vi "Autonomous Independent.vi"   [LabVIEW 2019]
doc: "This VI is called when autonomous begins, and will automatically be terminated when autonomous ends. You can carry out timed or sensor driven robot movement independently without needing to return to the caller."
uses:
  <vilib>/Rock Robotics/WPI/Utilities/WPI_GetSetVariantRefNum.vi
  <vilib>/Rock Robotics/Network Tables/NT Read String.vi
  <vilib>/Rock Robotics/Network Tables/NT Write Numeric Array.vi
panel:
  # "Be sure to right-click and choose Data Operations>>Make Current Value default if you want to save the array values with the VI"
types:
  T1 = typedef "WPI_JoystickDevRef.ctl" = cluster{"Device":T2}
  T2 = typedef "WPI_JoystickDeviceEnum.ctl" = enum16{"USB 0", "USB 1", "USB 2", "USB 3", "USB 4", "USB 5"}
  T3 = typedef "WPI_RobotDriveDevRef.ctl" = cluster{"DevStatus":errorcluster, "Motors[]":T4[], "Square Inputs":bool, "Max Output":dbl}
  T4 = typedef "WPI_MotorControlDeviceRef.ctl" = cluster{"DeviceStatus":errorcluster, "Type":T5, "PWM":cluster{"PWM Channel":T6, "DeadBand":T7}, "CAN":cluster{"Device Number":u8, "SetOutput VI Ref":variant, "GetOutput VI Ref":variant, "Enable VI Ref":variant, "Disable VI Ref":variant, "Data":variant}, "Invert":bool, "DIO PWM":cluster{"PWM \"Enable\" Channel":T6, "DIOChannel":T8, "PWM Rate":dbl}}
  T5 = typedef "WPI_MotorControlType.ctl" = enum16{"PWM", "CAN", "DIO PWM"}
  T6 = typedef "FPGA_DIOPWMChannel.ctl" = enum8{"PWM 0", "PWM 1", "PWM 2", "PWM 3", "PWM 4", "PWM 5", "PWM 6", "PWM 7", "PWM 8", "PWM 9", "PWM MXP 0", "PWM MXP 1", "PWM MXP 2", "PWM MXP 3", "PWM MXP 4", "PWM MXP 5", "PWM MXP 6", "PWM MXP 7", "PWM MXP 8", "PWM MXP 9", "Invalid"}
  T7 = typedef "WPI_PWMDeadband.ctl" = cluster{"Name":string, "maxPositivePwm":i32, "minPositivePwm":i32, "centerPwm":i32, "maxNegativePwm":i32, "minNegativePwm":i32, "angularRange":u16}
  T8 = typedef "FPGA_DIOChannel.ctl" = enum8{"DIO 0", "DIO 1", "DIO 2", "DIO 3", "DIO 4", "DIO 5", "DIO 6", "DIO 7", "DIO 8", "DIO 9", "DIO MXP 0", "DIO MXP 1", "DIO MXP 2", "DIO MXP 3", "DIO MXP 4", "DIO MXP 5", "DIO MXP 6", "DIO MXP 7", "DIO MXP 8", "DIO MXP 9", "DIO MXP 10", "DIO MXP 11", "DIO MXP 12", "DIO MXP 13", "DIO MXP 14", "DIO MXP 15", "SPI Port CS1", "SPI Port CS2", "SPI Port CS3", "SPI Port MISO", "SPI Port MOSI", "Invalid"}
  T9 = typedef "WPI_GyroDevRef.ctl" = cluster{"DevStatus":errorcluster, "Analog Channel":T10, "Gain (VoltsPerDegree/Second)":dbl, "Gyro Type":enum16{"Analog", "XRS450"}, "Handle":i32, "SPI Bus":T11, "Device Found":bool, "Sample Rate":dbl, "Calibrate On Open":bool, "Offset":dbl}
  T10 = typedef "FPGA_AIChannel.ctl" = enum8{"AI 0", "AI 1", "AI 2", "AI 3", "AI MXP 0", "AI MXP 1", "AI MXP 2", "AI MXP 3", "Invalid"}
  T11 = typedef "spi_bus.ctl" = enum16{"SPI On-Board, CS0", "SPI On-Board, CS1", "SPI On-Board, CS2", "SPI On-Board, CS3", "SPI MXP", "Invalid"}
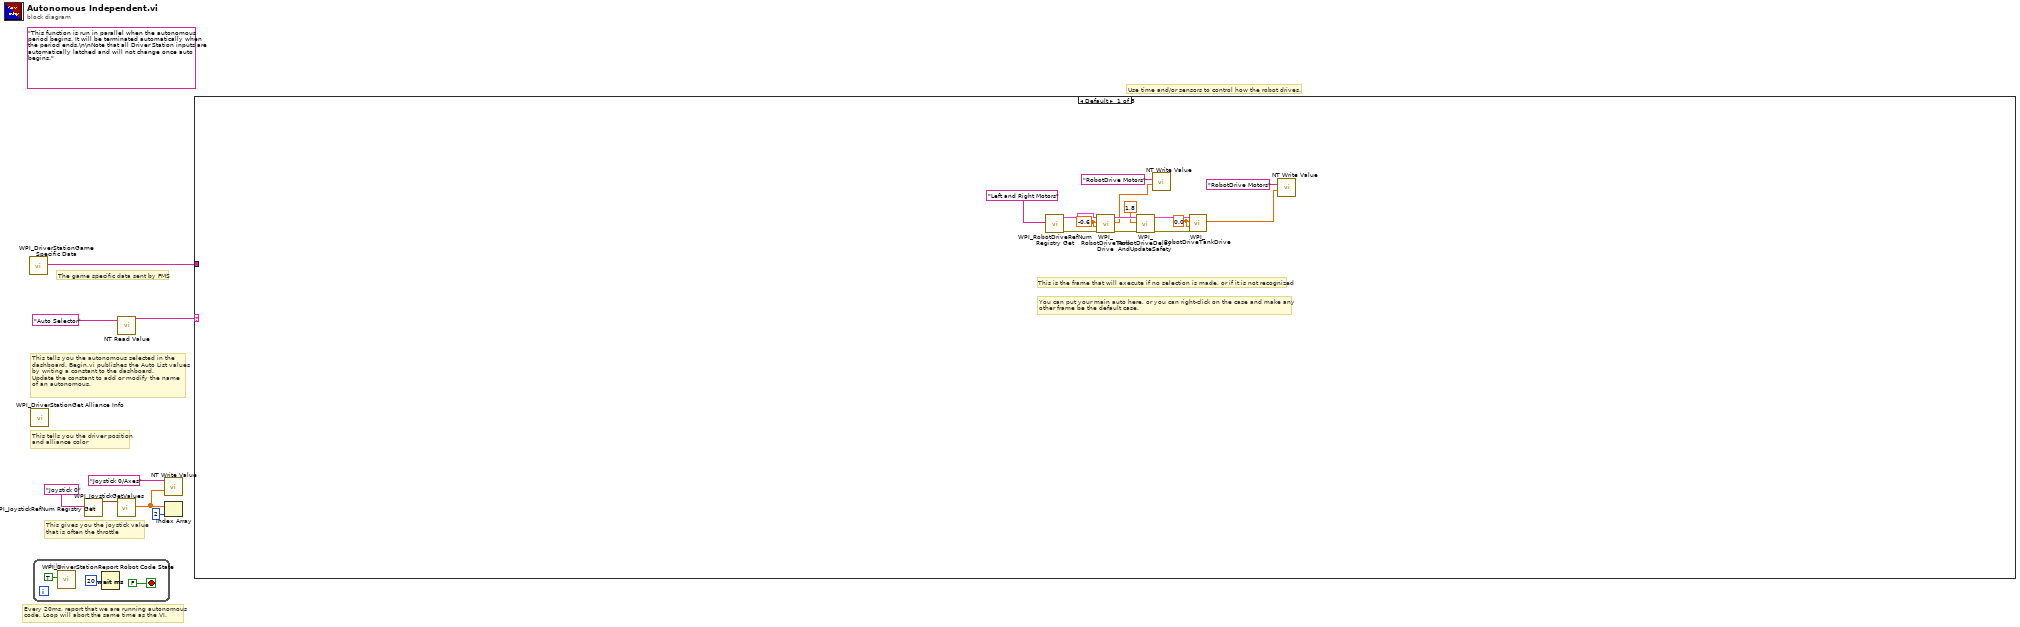
[diagram p0: block diagram]
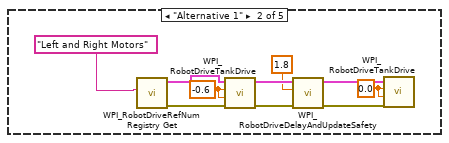
[diagram p2: hidden frame]
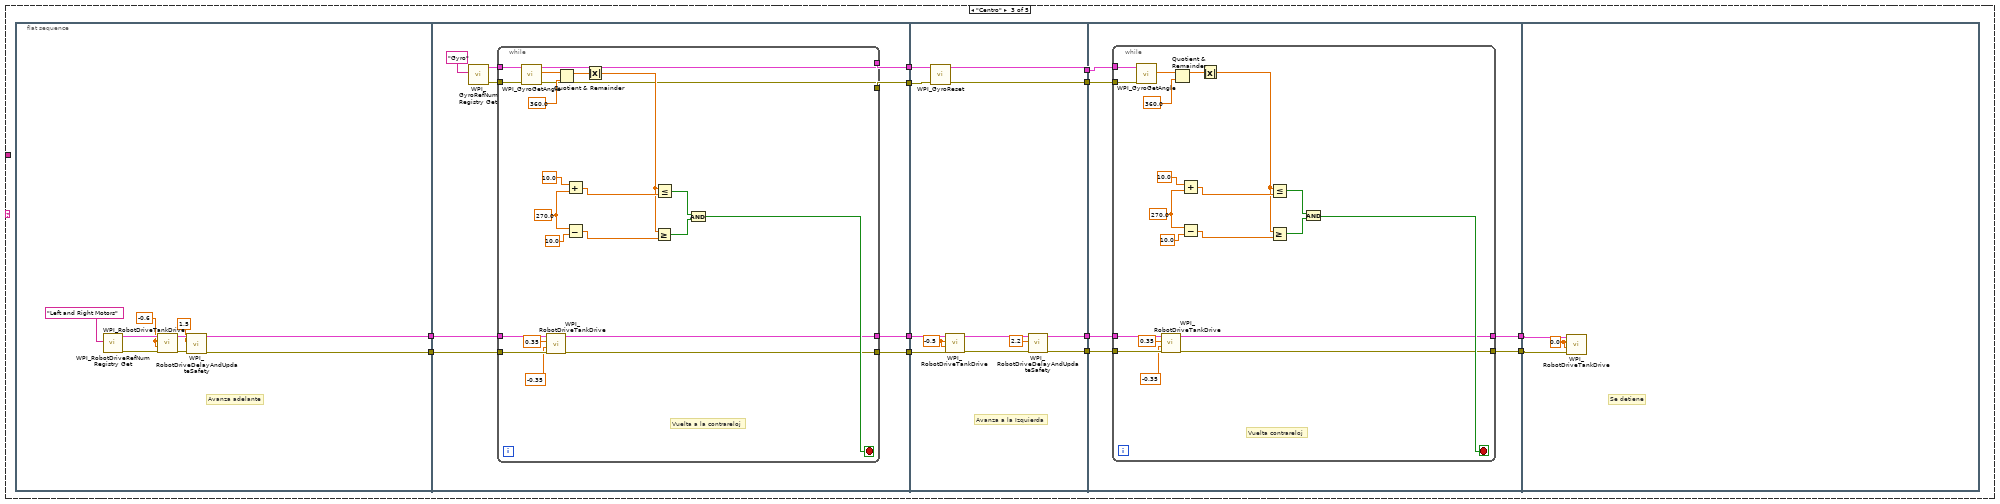
[diagram p3: hidden frame]
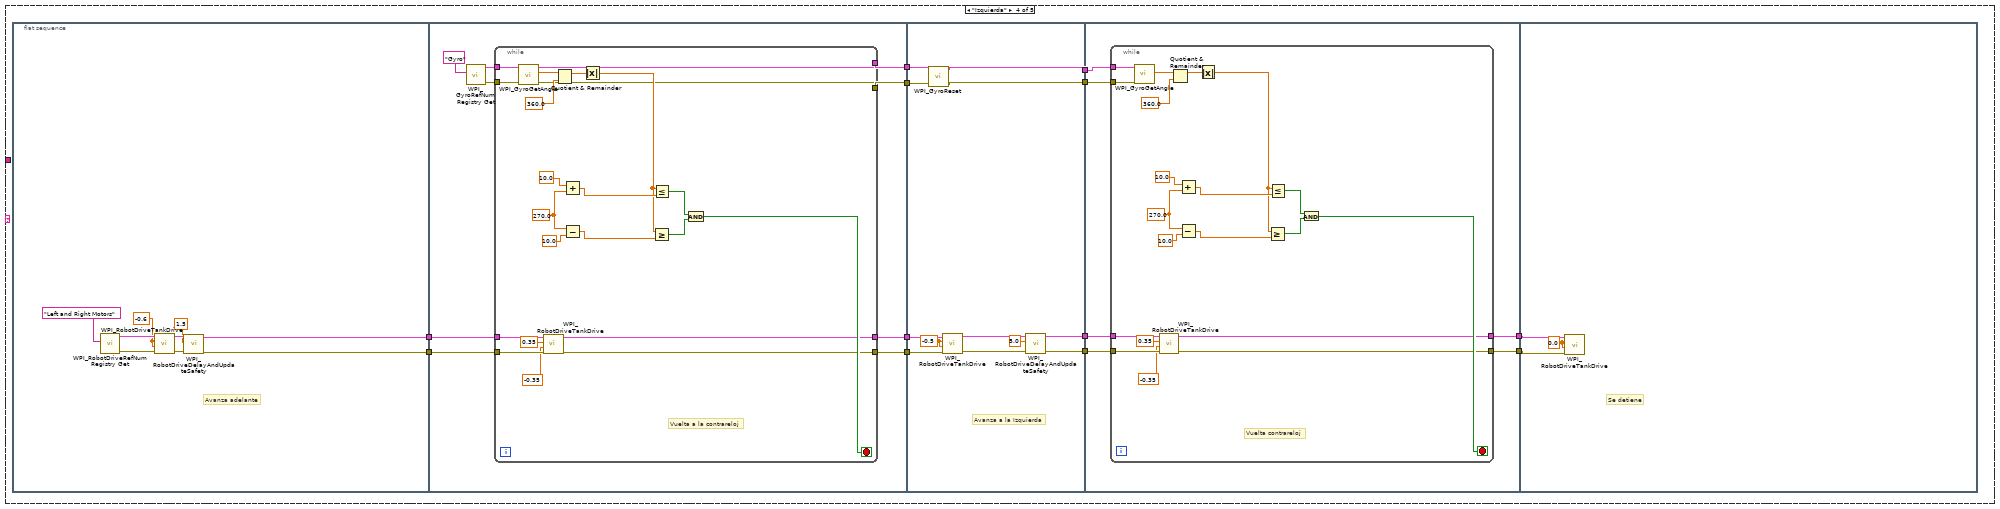
[diagram p4: hidden frame]
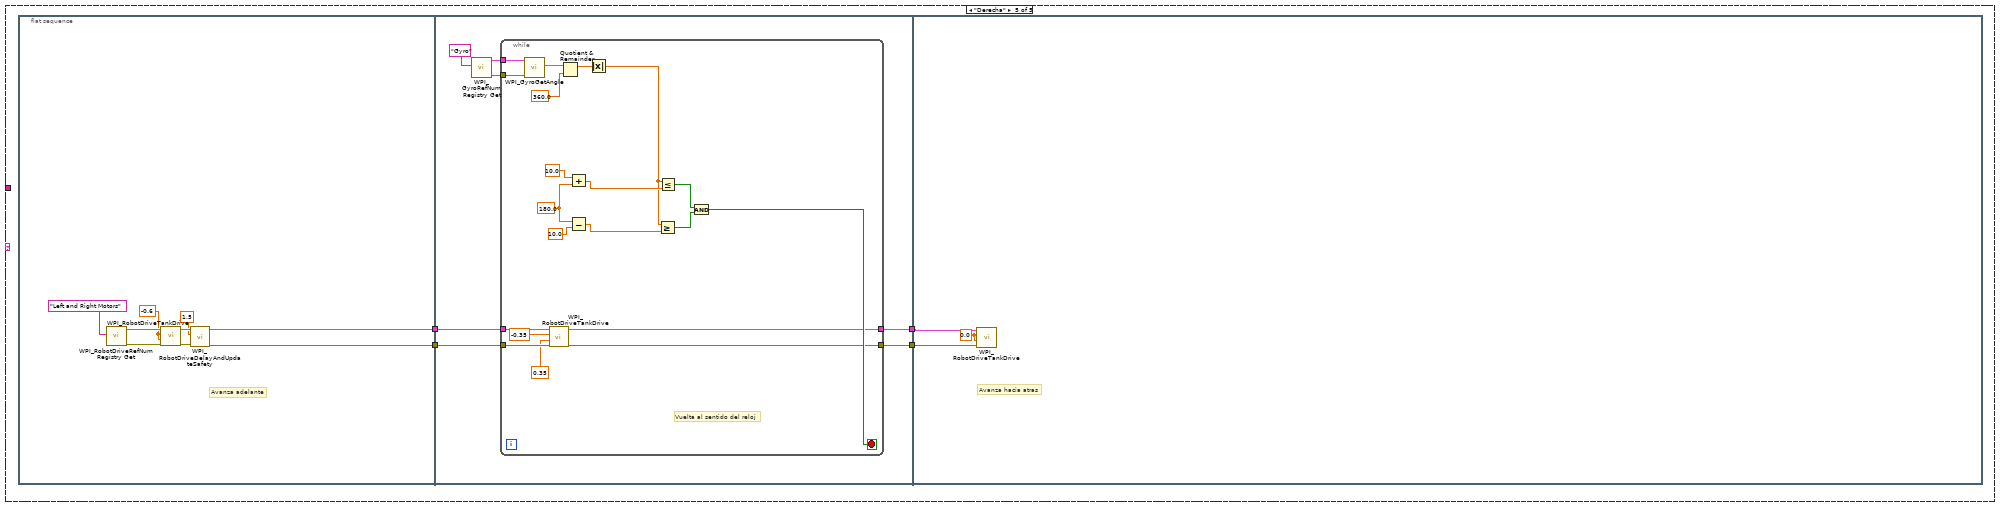
[diagram p5: hidden frame]
diagram:
  (unwired) "This function is run in parallel when the autonomous period begins. It will be terminated automatically when the period ends.\n\nNote that all Driver Station inputs are automatically latched and will not change once auto begins."
  # "The game specific data sent by FMS"
  # "This tells you the autonomous selected in the \ndashboard. Begin.vi publishes the Auto List values\nby writing a constant to the dashboard.\nUpdate the constant to add or modify the name\nof an autonomous."
  # "Every 20ms, report that we are running autonomous\ncode. Loop will abort the same time as the VI."
  # "This gives you the joystick value\nthat is often the throttle"
  # "Use time and/or sensors to control how the robot drives."
  # "This tells you the driver position\nand alliance color"
  n1 = call <vilib>:"WPI_DriverStationGame Specific Data.vi"() -> ("Game Specific Data"=w1:string)  [unwired: 11 in]
  n2 = call <vilib>:"WPI_DriverStationGet Alliance Info.vi"() -> ()  [unwired: 12 out]
  n3 = while {
    stop <- FALSE stop-if-true
    n4 = call <vilib>:"WPI_DriverStationReport Robot Code State.vi"("Autonomous"=TRUE) -> ()  [unwired: 10 in, 1 out]
    n5 = Wait (ms)(milliseconds to wait=u32 20) -> ()  [unwired: 1 out]
  }
  n6 = call <vilib>:"WPI_JoystickRefNum Registry Get.vi"("refnum name"="Joystick 0") -> ("JoystickDevRef"=w7:T1)  [unwired: 1 in, 9 out]
  n7 = call <vilib>:"WPI_JoystickGetValues.vi"("JoystickDevRef"=w7) -> ("Axes"=w3:dbl[])  [unwired: 6 in, 4 out]
  n8 = call-poly <vilib>:"NT Read Value.vi"("Name"="Auto Selector") -> ("String"=w4:string)  [unwired: 9 in, 1 out]
  n9 = call-poly <vilib>:"NT Write Value.vi"("Numeric Array"=w3, "Name"="Joystick 0/Axes") -> ()  [unwired: 9 in, 1 out]
  n10 = Index Array(array=w3, index=2) -> ()  [unwired: 1 out]
  n11 = case shown="Default" w4 {
    tunnel: w1 -> [_ _ _ _ _]
    frame Default {
      w16 = 0.0 ("Left axis value")
      w25 = -0.6 ("Left axis value")
      # "You can put your main auto here, or you can right-click on the case and make any\nother frame be the default case."
      # "This is the frame that will execute if no selection is made, or if it is not recognized"
      n12 = call <vilib>:"WPI_RobotDriveRefNum Registry Get.vi"("refnum name"="Left and Right Motors") -> ("error out"=w23:errorcluster, "RobotDriveDevRef"=w24:T3)  [unwired: 9 in]
      n13 = call <vilib>:"WPI_RobotDriveTankDrive.vi"("error in (no error)"=w23, "Right axis value"=w25, "Left axis value"=w25, "RobotDriveDevRef"=w24) -> ("error out"=w21:errorcluster, "Motor Values"=w13:dbl[], "RobotDriveDevRef"=w22:T3)  [unwired: 5 in]
      n14 = call <vilib>:"WPI_RobotDriveDelayAndUpdateSafety.vi"("error in (no error)"=w21, "Delay (s)"=1.8, "RobotDriveDevRef"=w22) -> ("error out"=w17:errorcluster, "RobotDriveDevRef 2"=w18:T3)  [unwired: 7 in]
      n15 = call-poly <vilib>:"NT Write Value.vi"("Numeric Array"=w13, "Name"="RobotDrive Motors") -> ()  [unwired: 9 in, 1 out]
      n16 = call <vilib>:"WPI_RobotDriveTankDrive.vi"("error in (no error)"=w17, "Right axis value"=w16, "Left axis value"=w16, "RobotDriveDevRef"=w18) -> ("Motor Values"=w12:dbl[])  [unwired: 5 in, 2 out]
      n17 = call-poly <vilib>:"NT Write Value.vi"("Numeric Array"=w12, "Name"="RobotDrive Motors") -> ()  [unwired: 9 in, 1 out]
    }
    frame "Alternative 1" {
      w26 = 0.0 ("Left axis value")
      w35 = -0.6 ("Left axis value")
      n18 = call <vilib>:"WPI_RobotDriveRefNum Registry Get.vi"("refnum name"="Left and Right Motors") -> ("error out"=w33:errorcluster, "RobotDriveDevRef"=w34:T3)  [unwired: 9 in]
      n19 = call <vilib>:"WPI_RobotDriveTankDrive.vi"("error in (no error)"=w33, "Right axis value"=w35, "Left axis value"=w35, "RobotDriveDevRef"=w34) -> ("error out"=w31:errorcluster, "RobotDriveDevRef"=w32:T3)  [unwired: 5 in, 1 out]
      n20 = call <vilib>:"WPI_RobotDriveDelayAndUpdateSafety.vi"("error in (no error)"=w31, "Delay (s)"=1.8, "RobotDriveDevRef"=w32) -> ("error out"=w27:errorcluster, "RobotDriveDevRef 2"=w28:T3)  [unwired: 7 in]
      n21 = call <vilib>:"WPI_RobotDriveTankDrive.vi"("error in (no error)"=w27, "Right axis value"=w26, "Left axis value"=w26, "RobotDriveDevRef"=w28) -> ()  [unwired: 5 in, 3 out]
    }
    frame "Centro" {
      n22 = flat-sequence {
        tunnel: [w49] -> w47
        tunnel: [w48] -> w46
        tunnel: w47 -> [w62]
        tunnel: w46 -> [w61]
        tunnel: [w60] -> w45
        tunnel: [w59] -> w44
        tunnel: [w58] -> w43
        tunnel: [w57] -> w42
        tunnel: w45 -> [w99]
        tunnel: w44 -> [w98]
        tunnel: [w93] -> w41
        tunnel: [w92] -> w40
        tunnel: w43 -> [w91]
        tunnel: w42 -> [w90]
        tunnel: [w89] -> w39
        tunnel: [w88] -> w38
        tunnel: w41 -> [w105]
        tunnel: w40 -> [w104]
        tunnel: w39 -> [w103]
        tunnel: w38 -> [w102]
        tunnel: [w101] -> w37
        tunnel: [w100] -> w36
        tunnel: w37 -> [w127]
        tunnel: w36 -> [w126]
        frame #0 {
          w53 = -0.6 ("Right axis value")
          # "Avanza adelante"
          n23 = call <vilib>:"WPI_RobotDriveRefNum Registry Get.vi"("refnum name"="Left and Right Motors") -> ("error out"=w55:errorcluster, "RobotDriveDevRef"=w54:T3)  [unwired: 9 in]
          n24 = call <vilib>:"WPI_RobotDriveTankDrive.vi"("error in (no error)"=w55, "Right axis value"=w53, "Left axis value"=w53, "RobotDriveDevRef"=w54) -> ("error out"=w52:errorcluster, "RobotDriveDevRef"=w51:T3)  [unwired: 5 in, 1 out]
          n25 = call <vilib>:"WPI_RobotDriveDelayAndUpdateSafety.vi"("error in (no error)"=w52, "Delay (s)"=1.5, "RobotDriveDevRef"=w51) -> ("error out"=w48:errorcluster, "RobotDriveDevRef 2"=w49:T3)  [unwired: 7 in]
        }
        frame #1 {
          n26 = call <vilib>:"WPI_GyroRefNum Registry Get.vi"("refnum name"="Gyro") -> ("error out"=w64:errorcluster, "GyroDevRef"=w63:T9)  [unwired: 9 in]
          n27 = while {
            tunnel: w64 -> [w84]
            tunnel: w63 -> [w83]
            tunnel: w62 -> [w81]
            tunnel: w61 -> [w82]
            tunnel: [w69] -> w60
            tunnel: [w68] -> w59
            tunnel: [w67] -> w58
            tunnel: [w66] -> w57
            stop <- w70 stop-if-true
            w77 = 270.0 ("y")
            # "Vuelta a la contrareloj"
            n28 = call <vilib>:"WPI_GyroGetAngle.vi"("error in"=w84, "GyroDevRef"=w83) -> ("error out"=w66:errorcluster, "Angle"=w87:dbl, "GyroDevRef"=w67:T9)  [unwired: 5 in, 2 out]
            n29 = call <vilib>:"WPI_RobotDriveTankDrive.vi"("error in (no error)"=w82, "Right axis value"=-0.35, "Left axis value"=0.35, "RobotDriveDevRef"=w81) -> ("error out"=w68:errorcluster, "RobotDriveDevRef"=w69:T3)  [unwired: 5 in, 1 out]
            n30 = Quotient & Remainder(x=w87, y=360.0) -> (x-y*floor(x/y)=w85:dbl)  [unwired: 1 out]
            n31 = Add(x=10.0, y=w77) -> (x+y=w75:dbl)
            n32 = Subtract(x=w77, y=10.0) -> (x-y=w74:dbl)
            n33 = Absolute Value(x=w85) -> (abs(x)=w71:dbl)
            n34 = Greater Or Equal?(x=w71, y=w74) -> (x >= y?=w72:bool)
            n35 = Less Or Equal?(x=w71, y=w75) -> (x <= y?=w73:bool)
            n36 = And(x=w73, y=w72) -> (x .and. y?=w70:bool)
          }
        }
        frame #2 {
          w97 = -0.5 ("Left axis value")
          # "Avanza a la Izquierda"
          n37 = call <vilib>:"WPI_GyroReset.vi"("error in"=w90, "GyroDevRef"=w91) -> ("error out"=w88:errorcluster, "GyroDevRef"=w89:T9)  [unwired: 8 in]
          n38 = call <vilib>:"WPI_RobotDriveTankDrive.vi"("error in (no error)"=w98, "Right axis value"=w97, "Left axis value"=w97, "RobotDriveDevRef"=w99) -> ("error out"=w95:errorcluster, "RobotDriveDevRef"=w96:T3)  [unwired: 5 in, 1 out]
          n39 = call <vilib>:"WPI_RobotDriveDelayAndUpdateSafety.vi"("error in (no error)"=w95, "Delay (s)"=2.2, "RobotDriveDevRef"=w96) -> ("error out"=w92:errorcluster, "RobotDriveDevRef 2"=w93:T3)  [unwired: 7 in]
        }
        frame #3 {
          n40 = while {
            tunnel: w102 -> [w122]
            tunnel: w103 -> [w121]
            tunnel: w105 -> [w119]
            tunnel: w104 -> [w120]
            tunnel: [w107] -> w101
            tunnel: [w106] -> w100
            stop <- w108 stop-if-true
            w115 = 270.0 ("y")
            # "Vuelta contrareloj"
            n41 = call <vilib>:"WPI_GyroGetAngle.vi"("error in"=w122, "GyroDevRef"=w121) -> ("Angle"=w125:dbl)  [unwired: 5 in, 4 out]
            n42 = call <vilib>:"WPI_RobotDriveTankDrive.vi"("error in (no error)"=w120, "Right axis value"=-0.35, "Left axis value"=0.35, "RobotDriveDevRef"=w119) -> ("error out"=w106:errorcluster, "RobotDriveDevRef"=w107:T3)  [unwired: 5 in, 1 out]
            n43 = Quotient & Remainder(x=w125, y=360.0) -> (x-y*floor(x/y)=w123:dbl)  [unwired: 1 out]
            n44 = Add(x=10.0, y=w115) -> (x+y=w113:dbl)
            n45 = Subtract(x=w115, y=10.0) -> (x-y=w112:dbl)
            n46 = Absolute Value(x=w123) -> (abs(x)=w109:dbl)
            n47 = Greater Or Equal?(x=w109, y=w112) -> (x >= y?=w110:bool)
            n48 = Less Or Equal?(x=w109, y=w113) -> (x <= y?=w111:bool)
            n49 = And(x=w111, y=w110) -> (x .and. y?=w108:bool)
          }
        }
        frame #4 {
          w128 = 0.0 ("Left axis value")
          # "Se detiene"
          n50 = call <vilib>:"WPI_RobotDriveTankDrive.vi"("error in (no error)"=w126, "Right axis value"=w128, "Left axis value"=w128, "RobotDriveDevRef"=w127) -> ()  [unwired: 5 in, 3 out]
        }
      }
    }
    frame "Izquierda" {
      n51 = flat-sequence {
        tunnel: [w142] -> w140
        tunnel: [w141] -> w139
        tunnel: w140 -> [w155]
        tunnel: w139 -> [w154]
        tunnel: [w153] -> w138
        tunnel: [w152] -> w137
        tunnel: [w151] -> w136
        tunnel: [w150] -> w135
        tunnel: w138 -> [w192]
        tunnel: w137 -> [w191]
        tunnel: [w186] -> w134
        tunnel: [w185] -> w133
        tunnel: w136 -> [w184]
        tunnel: w135 -> [w183]
        tunnel: [w182] -> w132
        tunnel: [w181] -> w131
        tunnel: w134 -> [w198]
        tunnel: w133 -> [w197]
        tunnel: w132 -> [w196]
        tunnel: w131 -> [w195]
        tunnel: [w194] -> w130
        tunnel: [w193] -> w129
        tunnel: w130 -> [w220]
        tunnel: w129 -> [w219]
        frame #0 {
          w146 = -0.6 ("Right axis value")
          # "Avanza adelante"
          n52 = call <vilib>:"WPI_RobotDriveRefNum Registry Get.vi"("refnum name"="Left and Right Motors") -> ("error out"=w148:errorcluster, "RobotDriveDevRef"=w147:T3)  [unwired: 9 in]
          n53 = call <vilib>:"WPI_RobotDriveTankDrive.vi"("error in (no error)"=w148, "Right axis value"=w146, "Left axis value"=w146, "RobotDriveDevRef"=w147) -> ("error out"=w145:errorcluster, "RobotDriveDevRef"=w144:T3)  [unwired: 5 in, 1 out]
          n54 = call <vilib>:"WPI_RobotDriveDelayAndUpdateSafety.vi"("error in (no error)"=w145, "Delay (s)"=1.5, "RobotDriveDevRef"=w144) -> ("error out"=w141:errorcluster, "RobotDriveDevRef 2"=w142:T3)  [unwired: 7 in]
        }
        frame #1 {
          n55 = call <vilib>:"WPI_GyroRefNum Registry Get.vi"("refnum name"="Gyro") -> ("error out"=w157:errorcluster, "GyroDevRef"=w156:T9)  [unwired: 9 in]
          n56 = while {
            tunnel: w157 -> [w177]
            tunnel: w156 -> [w176]
            tunnel: w155 -> [w174]
            tunnel: w154 -> [w175]
            tunnel: [w162] -> w153
            tunnel: [w161] -> w152
            tunnel: [w160] -> w151
            tunnel: [w159] -> w150
            stop <- w163 stop-if-true
            w170 = 270.0 ("y")
            # "Vuelta a la contrareloj"
            n57 = call <vilib>:"WPI_GyroGetAngle.vi"("error in"=w177, "GyroDevRef"=w176) -> ("error out"=w159:errorcluster, "Angle"=w180:dbl, "GyroDevRef"=w160:T9)  [unwired: 5 in, 2 out]
            n58 = call <vilib>:"WPI_RobotDriveTankDrive.vi"("error in (no error)"=w175, "Right axis value"=-0.35, "Left axis value"=0.35, "RobotDriveDevRef"=w174) -> ("error out"=w161:errorcluster, "RobotDriveDevRef"=w162:T3)  [unwired: 5 in, 1 out]
            n59 = Quotient & Remainder(x=w180, y=360.0) -> (x-y*floor(x/y)=w178:dbl)  [unwired: 1 out]
            n60 = Add(x=10.0, y=w170) -> (x+y=w168:dbl)
            n61 = Subtract(x=w170, y=10.0) -> (x-y=w167:dbl)
            n62 = Absolute Value(x=w178) -> (abs(x)=w164:dbl)
            n63 = Greater Or Equal?(x=w164, y=w167) -> (x >= y?=w165:bool)
            n64 = Less Or Equal?(x=w164, y=w168) -> (x <= y?=w166:bool)
            n65 = And(x=w166, y=w165) -> (x .and. y?=w163:bool)
          }
        }
        frame #2 {
          w190 = -0.5 ("Left axis value")
          # "Avanza a la Izquierda"
          n66 = call <vilib>:"WPI_GyroReset.vi"("error in"=w183, "GyroDevRef"=w184) -> ("error out"=w181:errorcluster, "GyroDevRef"=w182:T9)  [unwired: 8 in]
          n67 = call <vilib>:"WPI_RobotDriveTankDrive.vi"("error in (no error)"=w191, "Right axis value"=w190, "Left axis value"=w190, "RobotDriveDevRef"=w192) -> ("error out"=w188:errorcluster, "RobotDriveDevRef"=w189:T3)  [unwired: 5 in, 1 out]
          n68 = call <vilib>:"WPI_RobotDriveDelayAndUpdateSafety.vi"("error in (no error)"=w188, "Delay (s)"=5.0, "RobotDriveDevRef"=w189) -> ("error out"=w185:errorcluster, "RobotDriveDevRef 2"=w186:T3)  [unwired: 7 in]
        }
        frame #3 {
          n69 = while {
            tunnel: w195 -> [w215]
            tunnel: w196 -> [w214]
            tunnel: w198 -> [w212]
            tunnel: w197 -> [w213]
            tunnel: [w200] -> w194
            tunnel: [w199] -> w193
            stop <- w201 stop-if-true
            w208 = 270.0 ("y")
            # "Vuelta contrareloj"
            n70 = call <vilib>:"WPI_GyroGetAngle.vi"("error in"=w215, "GyroDevRef"=w214) -> ("Angle"=w218:dbl)  [unwired: 5 in, 4 out]
            n71 = call <vilib>:"WPI_RobotDriveTankDrive.vi"("error in (no error)"=w213, "Right axis value"=-0.35, "Left axis value"=0.35, "RobotDriveDevRef"=w212) -> ("error out"=w199:errorcluster, "RobotDriveDevRef"=w200:T3)  [unwired: 5 in, 1 out]
            n72 = Quotient & Remainder(x=w218, y=360.0) -> (x-y*floor(x/y)=w216:dbl)  [unwired: 1 out]
            n73 = Add(x=10.0, y=w208) -> (x+y=w206:dbl)
            n74 = Subtract(x=w208, y=10.0) -> (x-y=w205:dbl)
            n75 = Absolute Value(x=w216) -> (abs(x)=w202:dbl)
            n76 = Greater Or Equal?(x=w202, y=w205) -> (x >= y?=w203:bool)
            n77 = Less Or Equal?(x=w202, y=w206) -> (x <= y?=w204:bool)
            n78 = And(x=w204, y=w203) -> (x .and. y?=w201:bool)
          }
        }
        frame #4 {
          w221 = 0.0 ("Left axis value")
          # "Se detiene"
          n79 = call <vilib>:"WPI_RobotDriveTankDrive.vi"("error in (no error)"=w219, "Right axis value"=w221, "Left axis value"=w221, "RobotDriveDevRef"=w220) -> ()  [unwired: 5 in, 3 out]
        }
      }
    }
    frame "Derecha" {
      n80 = flat-sequence {
        tunnel: [w227] -> w225
        tunnel: [w226] -> w224
        tunnel: w225 -> [w238]
        tunnel: w224 -> [w237]
        tunnel: [w236] -> w223
        tunnel: [w235] -> w222
        tunnel: w223 -> [w263]
        tunnel: w222 -> [w262]
        frame #0 {
          w231 = -0.6 ("Right axis value")
          # "Avanza adelante"
          n81 = call <vilib>:"WPI_RobotDriveRefNum Registry Get.vi"("refnum name"="Left and Right Motors") -> ("error out"=w233:errorcluster, "RobotDriveDevRef"=w232:T3)  [unwired: 9 in]
          n82 = call <vilib>:"WPI_RobotDriveTankDrive.vi"("error in (no error)"=w233, "Right axis value"=w231, "Left axis value"=w231, "RobotDriveDevRef"=w232) -> ("error out"=w230:errorcluster, "RobotDriveDevRef"=w229:T3)  [unwired: 5 in, 1 out]
          n83 = call <vilib>:"WPI_RobotDriveDelayAndUpdateSafety.vi"("error in (no error)"=w230, "Delay (s)"=1.5, "RobotDriveDevRef"=w229) -> ("error out"=w226:errorcluster, "RobotDriveDevRef 2"=w227:T3)  [unwired: 7 in]
        }
        frame #1 {
          n84 = call <vilib>:"WPI_GyroRefNum Registry Get.vi"("refnum name"="Gyro") -> ("error out"=w240:errorcluster, "GyroDevRef"=w239:T9)  [unwired: 9 in]
          n85 = while {
            tunnel: w240 -> [w258]
            tunnel: w239 -> [w257]
            tunnel: w238 -> [w255]
            tunnel: w237 -> [w256]
            tunnel: [w243] -> w236
            tunnel: [w242] -> w235
            stop <- w244 stop-if-true
            w251 = 180.0 ("y")
            # "Vuelta al sentido del reloj"
            n86 = call <vilib>:"WPI_GyroGetAngle.vi"("error in"=w258, "GyroDevRef"=w257) -> ("Angle"=w261:dbl)  [unwired: 5 in, 4 out]
            n87 = call <vilib>:"WPI_RobotDriveTankDrive.vi"("error in (no error)"=w256, "Right axis value"=0.35, "Left axis value"=-0.35, "RobotDriveDevRef"=w255) -> ("error out"=w242:errorcluster, "RobotDriveDevRef"=w243:T3)  [unwired: 5 in, 1 out]
            n88 = Quotient & Remainder(x=w261, y=360.0) -> (x-y*floor(x/y)=w259:dbl)  [unwired: 1 out]
            n89 = Add(x=10.0, y=w251) -> (x+y=w249:dbl)
            n90 = Subtract(x=w251, y=10.0) -> (x-y=w248:dbl)
            n91 = Absolute Value(x=w259) -> (abs(x)=w245:dbl)
            n92 = Greater Or Equal?(x=w245, y=w248) -> (x >= y?=w246:bool)
            n93 = Less Or Equal?(x=w245, y=w249) -> (x <= y?=w247:bool)
            n94 = And(x=w247, y=w246) -> (x .and. y?=w244:bool)
          }
        }
        frame #2 {
          w264 = 0.0 ("Left axis value")
          # "Avanza hacia atras"
          n95 = call <vilib>:"WPI_RobotDriveTankDrive.vi"("error in (no error)"=w262, "Right axis value"=w264, "Left axis value"=w264, "RobotDriveDevRef"=w263) -> ()  [unwired: 5 in, 3 out]
        }
      }
    }
  }
